vi "Filter SRL Command to 19 bits.vi"(11 "SRL Command In":string) -> (3 "19-bit SRL Command":string)   [LabVIEW 2017, in "Host SRL.lvlib"]
uses:
  Host SRL.lvlib
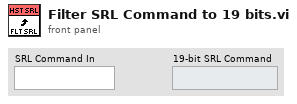
[diagram p1: front panel]
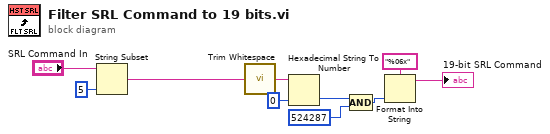
[diagram p0: block diagram]
diagram:
  n1 = String Subset(string="SRL Command In", length (rest)=5 ("length (rest)")) -> (substring=w1:string)  [unwired: 1 in]
  n2 = call <vilib>:"Trim Whitespace.vi"("string"=w1) -> ("trimmed string"=w2:string)  [unwired: 1 in]
  n3 = Hexadecimal String To Number(string=w2, default (0uL)=u32 0 ("default (0 U32)")) -> (number=w6:u32)  [unwired: 1 in, 1 out]
  n4 = Compound Arithmetic op=AND(w6, u32 524287 ("value")) -> (w7:u32)
  n5 = Format Into String(format string="%06x", w7) -> (resulting string=→"19-bit SRL Command":string)  [unwired: 2 in, 1 out]
